vi "Restore Plot Property.vi"(6 "Control Ref Queue":T1, 8 "error in (no error)":errorcluster, 11 "2D Plotmatrix.lvclass in":refnum<class "XY Plot Matrix.lvclass">) -> (0 "error out":errorcluster, 3 "2D Plotmatrix.lvclass out":refnum<class "XY Plot Matrix.lvclass">)   [LabVIEW 2017, in "XY Plot Matrix.lvclass"]
uses:
  <vilib>/Math Plots/2D Math Plots/XY Plot Matrix/XY Plot Matrix/XY Plot Matrix.lvclass
  <vilib>/Math Plots/2D Math Plots/2D Plot/Action String/XYPlotMatrix Ctrl Act Queue.ctl
  <vilib>/Math Plots/2D Math Plots/2D Plot/Action String/XYPlotMatrix Ctrl Act Cluster.ctl
  <vilib>/Math Plots/2D Math Plots/2D Plot/Action String/2DMathPlot State Class.ctl
  <vilib>/Math Plots/2D Math Plots/XY Plot Matrix/XY Plot Matrix/XY Plot Matrix.lvclass/XY Plot Matrix.ctl
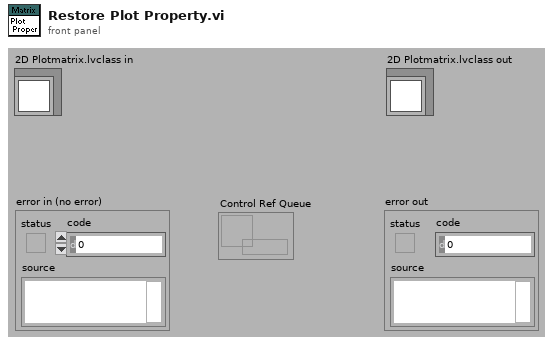
[diagram p1: front panel]
types:
  T1 = typedef "XYPlotMatrix Ctrl Act Queue.ctl" = refnum<queue>
  T2 = typedef "XYPlotMatrix Ctrl Act Cluster.ctl" = cluster{"Facade VI":refnum<vi>, "XControl":refnum<vi>, "Sub Panel":refnum<vi>, "Sub VI":refnum<vi>, "Export Image":refnum<vi>, "Display State Change Class":T3}
  T3 = typedef "2DMathPlot State Class.ctl" = enum16{"Update All (Undo)", "Update General", "Update Appearance", "Update Format", "Update Scale", "Update Marker", "Update Cursor", "None"}
  T4 = typedef "XY Plot Matrix.lvclass/Plotmatrix Property Array.ctl" = T5[][]
  T5 = typedef "XY Plot Matrix.lvclass/Plotmatrix Property.ctl" = cluster{"Plot Property Array":T6}
  T6 = typedef "2D Plot.lvclass/Plot Property Array.ctl" = T7[]
  T7 = typedef "2D Plot.lvclass/Plot Property.ctl" = cluster{"Bar Plot Style":u8, "DigitalLineStyle":u8, "TransitionLocation":u8, "Transition Type":u8, "Fill To":i16, "Fill/Pt. Color":u32, "Label Style":u8, "Line Style":u8, "Line Width":u8, "Plot Color":u32, "Plot Interpolation":u8, "Plot Name":string, "Point Style":u8, "Visible?":bool, "XScaleIdx":u32, "YScaleIdx":u32}
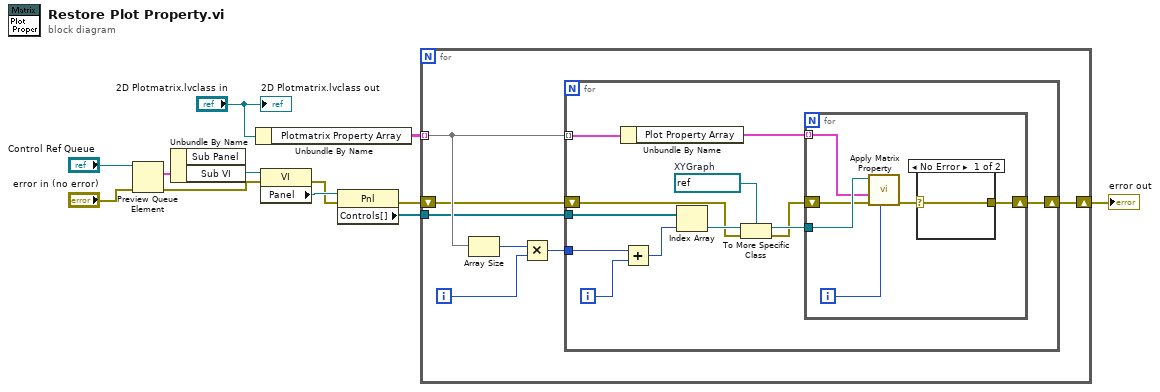
[diagram p0: block diagram]
diagram:
  n1 = Preview Queue Element(queue="Control Ref Queue", error in (no error)="error in (no error)") -> (element=w8:T2, error out=w5:errorcluster)  [unwired: 3 out]
  n2 = Unbundle By Name(w8) -> ("Sub VI"=w7:refnum<vi>)  [unwired: 1 out]
  n3 = Unbundle By Name("2D Plotmatrix.lvclass in") -> ("Plotmatrix Property Array"=w2:T4)
  n4 = property class="VI"(reference=w7, error in=w5) -> (error out=w10:errorcluster, "Panel"=w11:refnum<vi>)  [unwired: 1 out]
  n5 = property class="Pnl"(reference=w11, error in=w10) -> (error out=w3:errorcluster, "Controls[]"=w4:refnum<vi>[])  [unwired: 1 out]
  n6 = for {
    tunnel: w2 -> [w18] mode=indexing
    tunnel: w4 -> [w15]
    shift-right: [w13] -> w1
    shift-left: w3 -> [w14]
    i -> [w19]
    n7 = Array Size(array=w18) -> (size(s)=w17:i32)
    n8 = Multiply(x=w17, y=w19) -> (x*y=w16:i32)
    n9 = for {
      tunnel: w18 -> [w21] mode=indexing
      tunnel: w16 -> [w30]
      tunnel: w15 -> [w29]
      shift-right: [w22] -> w13
      shift-left: w14 -> [w23]
      i -> [w31]
      w27 = refnum<vi> refnum  # XYGraph
      n10 = Unbundle By Name(w21) -> ("Plot Property Array"=w20:T6)
      n11 = Add(x=w30, y=w31) -> (x+y=w28:i32)
      n12 = Index Array(array=w29, index=w28) -> (element=w26:refnum<vi>)
      n13 = To More Specific Class(target class=w27, reference=w26, error in=w23) -> (specific class reference=w25:refnum<vi>, error out=w24:errorcluster)
      n14 = for {
        tunnel: w25 -> [w37]
        tunnel: w20 -> [w32] mode=indexing
        shift-right: [w34] -> w22
        shift-left: w24 -> [w36]
        i -> [w33]
        n15 = call <vilib>:"Apply Matrix Property.vi"("Plot ID"=w33, "error in (no error)"=w36, "Plot Property"=w32, "Polar Area Ref In"=w37) -> ("error out"=w35:errorcluster)  [unwired: 7 out]
        n16 = case shown="No Error" w35 {
          selector: w35 -> [w38 _]
          tunnel: [w38 _] -> w34
          frame No Error {
          }
          frame Error {
          }
        }
      }
    }
  }
  "error out" <- w1
  "2D Plotmatrix.lvclass out" <- "2D Plotmatrix.lvclass in"
